vi "Main.vi"() -> ()   [LabVIEW 2020]
panel:
  out "error":errorcluster
  in  "Add Page":bool
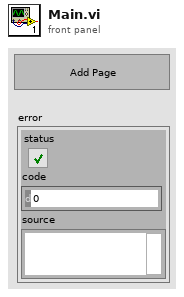
[diagram p1: front panel]
types:
  T1 = enum32{"Invalid", "Standard", "Closed", "Hidden", "Minimized", "Maximized"}
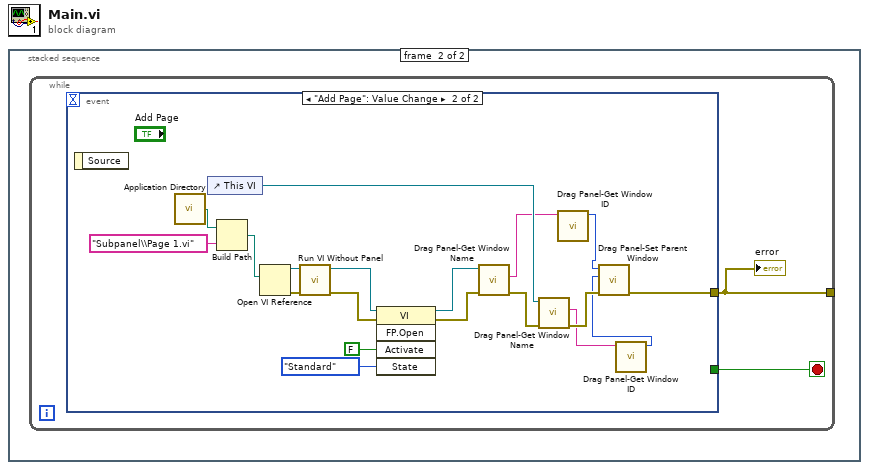
[diagram p0: block diagram]
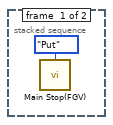
[diagram p2: hidden frame]
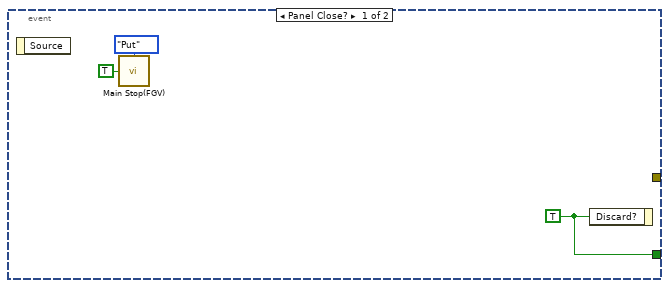
[diagram p3: hidden frame]
diagram:
  n1 = stacked-sequence {
    frame #0 {
      n2 = call "Main Stop(FGV).vi"("Method"=enum16{"Get", "Put"}."Put") -> ()  [unwired: 3 in, 1 out]
    }
    frame #1 {
      n3 = while {
        tunnel: [w2] -> _
        stop <- w3 stop-if-true
        n4 = event shown="[1] \"Add Page\": Value Change" {
          selector: _ -> [_ _]
          dyn-events: _ -> [_ _]
          timeout: _ -> [_ _]
          tunnel: [w6 _] -> w3
          tunnel: [_ w17] -> w2
          event Panel Close? {
            w6 = TRUE ("Discard?")
            n5 = event-data() -> ()  [unwired: 1 in, 1 out]
            n6 = call "Main Stop(FGV).vi"("Method"=enum16{"Get", "Put"}."Put", "Stop In"=TRUE) -> ()  [unwired: 2 in, 1 out]
            n7 = event-data("Discard?"=w6) -> ()  [unwired: 1 in, 1 out]
          }
          event "Add Page": Value Change {
            n8 = event-data() -> ()  [unwired: 1 in, 1 out]
            n9 = call <vilib>:"Application Directory.vi"() -> ("Application Directory"=w24:path)
            n10 = control-ref of="This VI"() -> (w22:refnum<vi>)
            n11 = Build Path(base path=w24, name or relative path="Subpanel\\Page 1.vi") -> (appended path=w23:path)
            n12 = Open VI Reference(vi path=w23) -> (vi reference=w19:refnum<vi>, error out=w20:errorcluster)  [unwired: 5 in]
            n13 = call "Run VI Without Panel.vi"("error in"=w20, "VI Reference"=w19) -> ("error out"=w14:errorcluster, "vi reference"=w12:refnum<vi>)  [unwired: 8 in]
            n14 = invoke class="VI" method="FP.Open"(reference=w12, error in=w14, "Activate"=FALSE ("Activate?"), "State"=T1."Standard") -> (reference out=w11:refnum<vi>, error out=w13:errorcluster)  [unwired: 1 in, 3 out]
            n15 = call "Drag Panel-Get Window Name.vi"("error in"=w13, "VI Refnum In"=w11) -> ("error out"=w21:errorcluster, "Window Name"=w10:string)  [unwired: 7 in, 1 out]
            n16 = call "Drag Panel-Get Window Name.vi"("error in"=w21, "VI Refnum In"=w22) -> ("error out"=w18:errorcluster, "Window Name"=w8:string)  [unwired: 7 in, 1 out]
            n17 = call "Drag Panel-Get Window ID.vi"("Window Name"=w10) -> ("Window ID"=w9:u32)  [unwired: 9 in, 1 out]
            n18 = call "Drag Panel-Get Window ID.vi"("Window Name"=w8) -> ("Window ID"=w7:u32)  [unwired: 9 in, 1 out]
            n19 = call "Drag Panel-Set Parent Window.vi"("error in"=w18, "Parent Window ID"=w7, "Child Window ID"=w9) -> ("error out"=w17:errorcluster)  [unwired: 7 in, 1 out]
          }
        }
        "error" <- w2
      }
    }
  }
